vi "WheeTrometerChrom_2.vi"() -> ()   [LabVIEW 2020]
uses:
  <vilib>/Analysis/baseanly.llb/Mean (DBL).vi
  WheeChromGlobals.vi
  <vilib>/Instr/_visa.llb/VISA Configure Serial Port (Instr).vi
  <vilib>/Platform/NI_3dgraph.lvlib
  <vilib>/Analysis/NI_AALBase.lvlib
panel:
  in  "Auto Find 2":bool=TRUE
  out "Connection":bool
  in  "Tab Control":enum32{"Chrom Data", "Spectrometer Settings"}(tab)=enum."Spectrometer Settings"
  in  "3D Surface":refnum<k7>(container)
  out "Latest Spectrum":cluster{"WavelengthCal":dbl[], "Array":i32[]}(graph)
  out "Chromatogram at wavelength of interest":i32[](graph)
  in  "Start":bool
  in  "Length of Chromatogram (sec)":dbl=120.0
  in  "Wavelength of Interest (nm)":dbl=500.0
  in  "Date file path":path
  out "XY Graph":cluster{"WavelengthCal":dbl[], "Array":i32[]}(graph)
  in  "Single Spec":bool
  in  "spectra to average (per spec)":dbl=1.0
  in  "pixels to average (per spec)":dbl=2.0
  in  "Intergratin time (ms) (per spec)":dbl=2.0
  in  "Initiate":bool
  out "Connected on COM port:":refnum<visa-resource-name>="COM7"
  out "A":dbl=249.12
  out "B":dbl=0.14952
  out "C":dbl=32.477
  out "+":dbl=100.0
  out "=":dbl=125.0
  in  "Auto Find":bool=TRUE
  in  "reference":refnum<visa-resource-name>
  # "f = sin(pi*i/sizeOfdata);\n   wavelengthI(i)= A+h*B+C*f;"
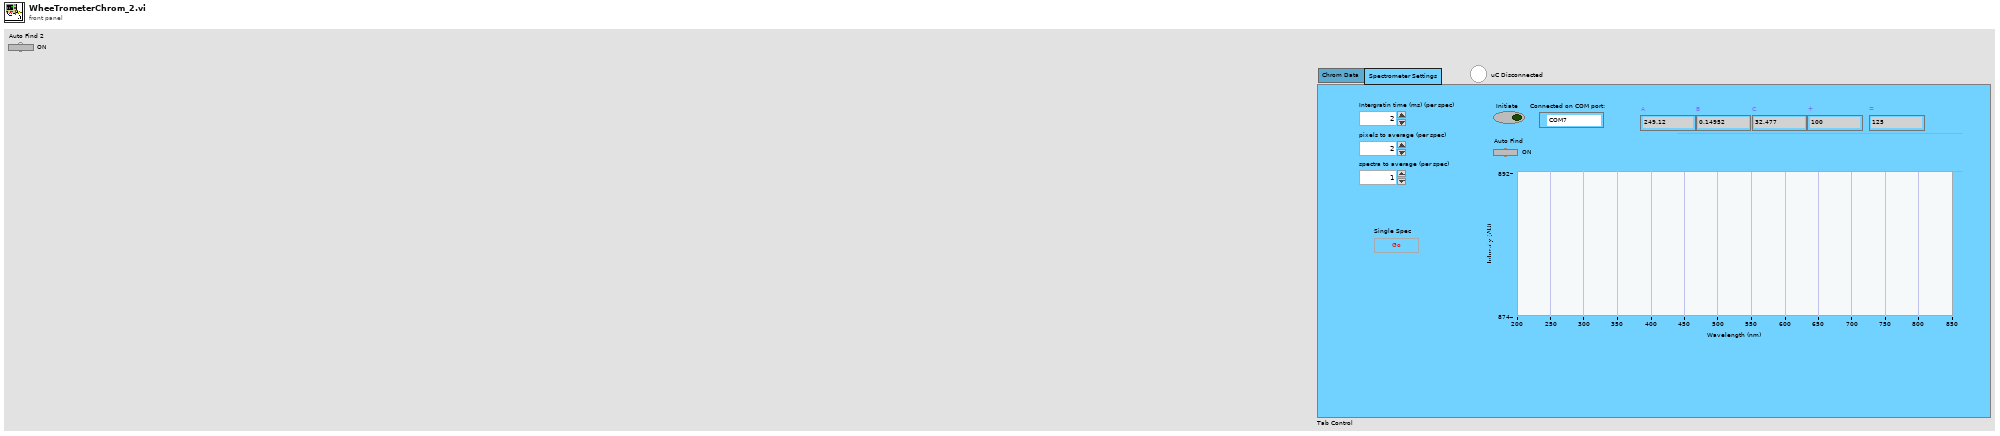
[diagram p1: front panel]
types:
  T1 = enum16{"open", "replace", "create", "open or create", "replace or create", "replace or create with confirmation"}
  T2 = enum16{"open", "open or create", "create or replace", "create", "open (read-only)"}
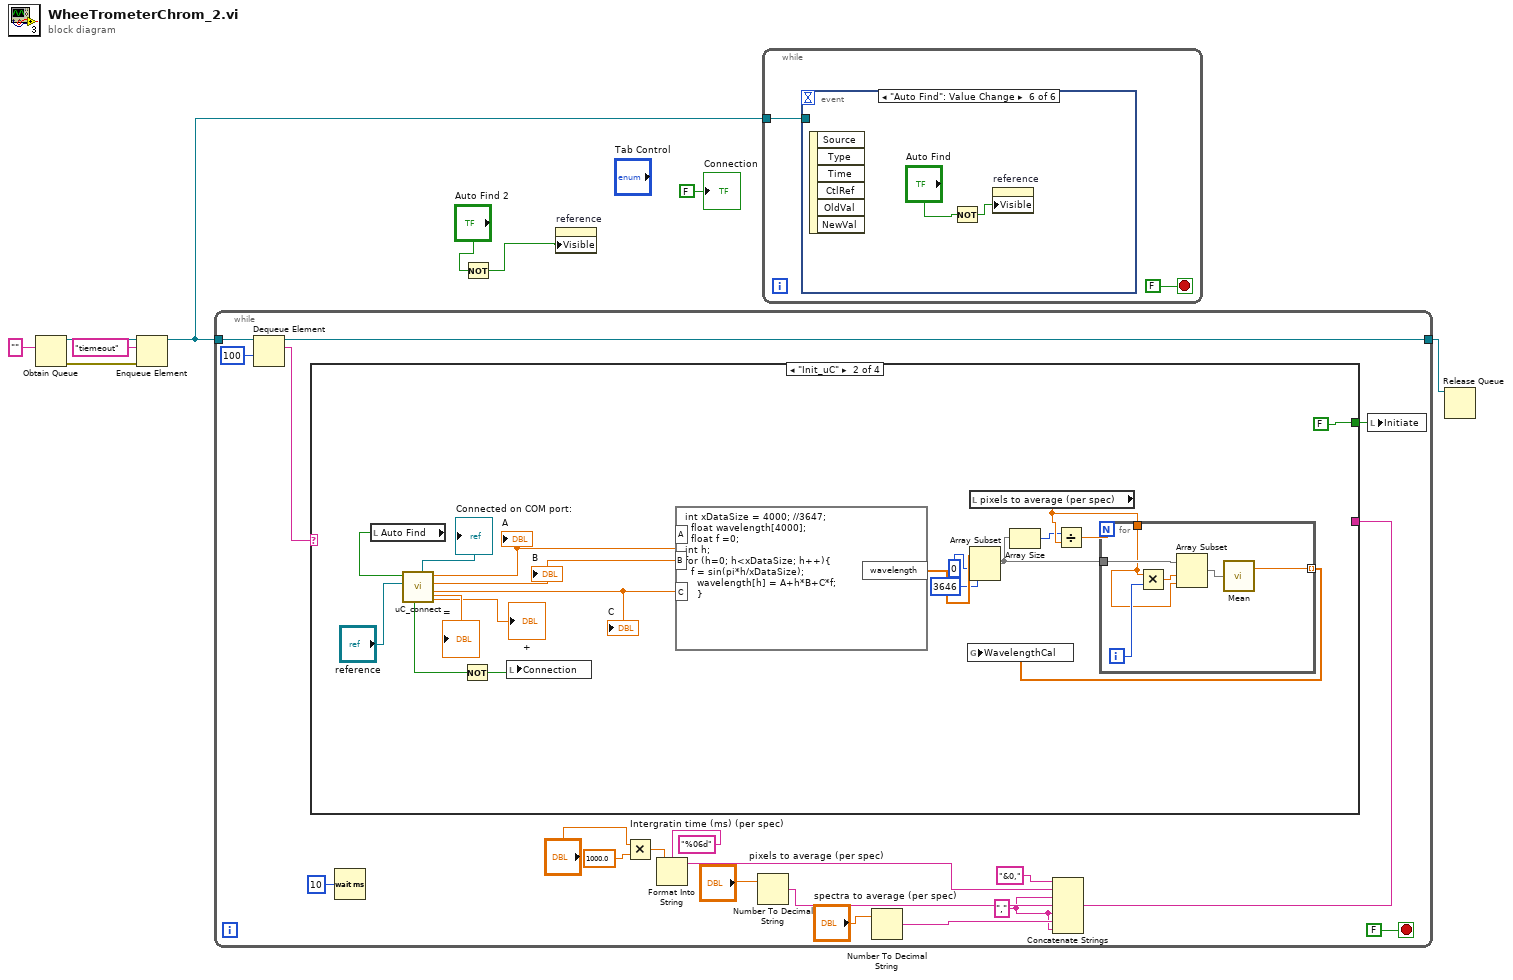
[diagram p0: block diagram]
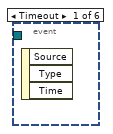
[diagram p2: hidden frame]
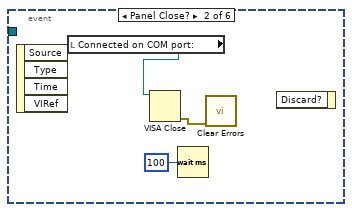
[diagram p3: hidden frame]
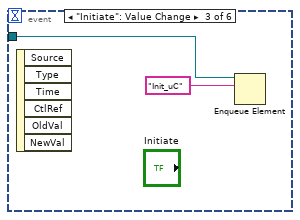
[diagram p4: hidden frame]
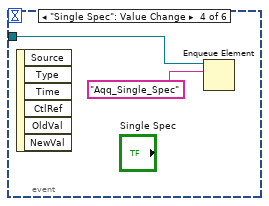
[diagram p5: hidden frame]
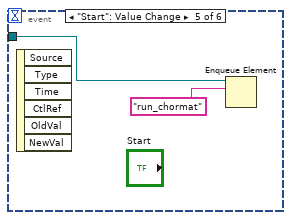
[diagram p6: hidden frame]
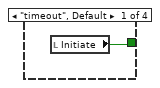
[diagram p7: hidden frame]
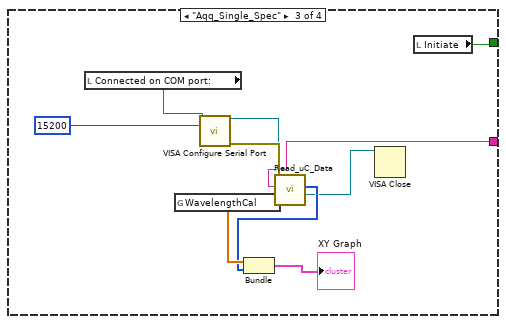
[diagram p8: hidden frame]
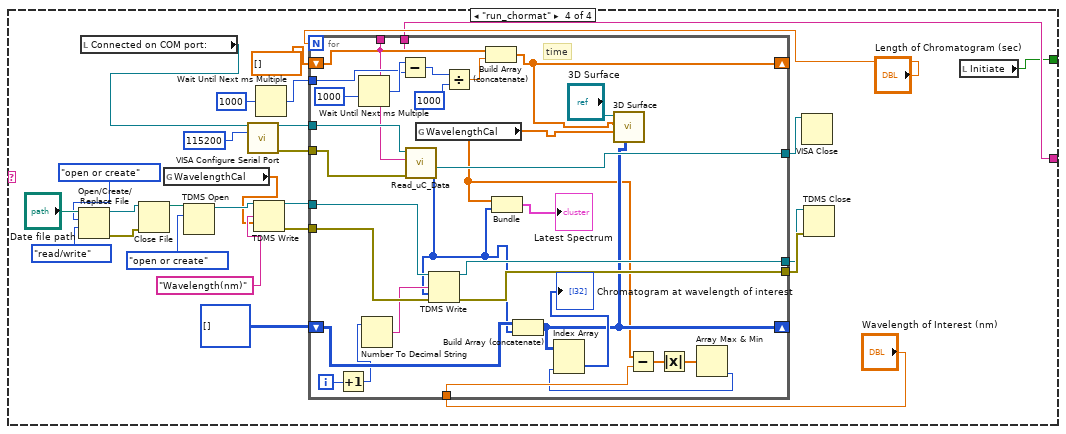
[diagram p9: hidden frame]
diagram:
  n1 = Obtain Queue(element data type="") -> (queue out=w7:refnum<queue>, error out=w5:errorcluster)  [unwired: 4 in, 1 out]
  n2 = Enqueue Element(queue=w7, element="tiemeout", error in (no error)=w5) -> (queue out=w3:refnum<queue>)  [unwired: 1 in, 2 out]
  n3 = while {
    tunnel: w3 -> [w27]
    tunnel: [w26] -> w4
    stop <- FALSE stop-if-true
    w15 = "," ("string")
    n4 = Dequeue Element(queue=w27, timeout in ms (-1)=100) -> (queue out=w26:refnum<queue>, element=w25:string)  [unwired: 1 in, 2 out]
    n5 = Wait (ms)(milliseconds to wait=u32 10) -> ()  [unwired: 1 out]
    n6 = Multiply(x="Intergratin time (ms) (per spec)", y=1000.0) -> (x*y=w17:dbl)
    n7 = Format Into String(format string="%06d", w17) -> (resulting string=w21:string)  [unwired: 2 in, 1 out]
    n8 = Number To Decimal String(number="pixels to average (per spec)") -> (decimal integer string=w22:string)  [unwired: 1 in]
    n9 = Number To Decimal String(number="spectra to average (per spec)") -> (decimal integer string=w23:string)  [unwired: 1 in]
    n10 = Concatenate Strings("&0," ("string"), w21, w15, w22, w15, w23, w15) -> (w12:string)
    n11 = case shown="\"Init_uC\"" w25 {
      tunnel: w12 -> [_ _ w57 w71]
      tunnel: [w29 FALSE ("Initiate") w55 w70] -> w10
      frame "timeout", Default {
        n12 = local read "Initiate"() -> (w29:bool)
      }
      frame "Init_uC" {
        n13 = local read "Auto Find"() -> (w32:bool)
        n14 = call "uC_connect.vi"("reference"="reference", "find port"=w32) -> ("+"=→"+":dbl, "C"=w39:dbl, "B"=w38:dbl, "A"=w37:dbl, "="=→"=":dbl, "VISA resource name out"=→"Connected on COM port:":refnum<visa-resource-name>, "status"=w48:bool)  [unwired: 2 in, 1 out]
        "A" <- w37
        "B" <- w38
        "C" <- w39
        n15 = Not(x=w48) -> (.not. x?=w47:bool)
        n16 = local write "Connection"(w47) -> ()
        n17 = formula code="int xDataSize = 4000; //3647;                \n  float wavelength[4000];\n  float f =0;\nint h;\nfor (h=0; h<xDataSize; h++){\n  f = sin(pi*h/xDataSize);\n    wavelength[h] = A+h*B+C*f;\n    }"("A"=w37, "B"=w38, "C"=w39) -> ("wavelength"=w40:dbl[])
        n18 = local read "pixels to average (per spec)"() -> (w44:dbl)
        n19 = Array Subset(array=w40, index=0, length=3646) -> (w43:dbl[])
        n20 = Array Size(array=w43) -> (size(s)=w41:i32)
        n21 = Divide(x=w41, y=w44) -> (x/y=w42:dbl)
        n22 = for {
          N: w42 -> [_]
          tunnel: w43 -> [w54]
          tunnel: w44 -> [w51]
          tunnel: [w49] -> w45 mode=indexing
          i -> [w52]
          n23 = Multiply(x=w51, y=w52) -> (x*y=w53:dbl)
          n24 = Array Subset(array=w54, index=w53, length=w51) -> (w50:dbl[])
          n25 = call-poly <vilib>:"Mean.vi"("X"=w50) -> ("mean"=w49:dbl)  [unwired: 1 out]
        }
        n26 = global write "WheeChromGlobals.vi" "WavelengthCal"(w45) -> ()
      }
      frame "Aqq_Single_Spec" {
        n27 = local read "Connected on COM port:"() -> (w58:refnum<visa-resource-name>)
        n28 = global read "WheeChromGlobals.vi" "WavelengthCal"() -> (w64:dbl[])
        n29 = call-poly "VISA Configure Serial Port"("VISA resource name"=w58, "baud rate (9600)"=u32 15200) -> ("VISA resource name out"=w59:refnum<visa-resource-name>, "error out"=w60:errorcluster)  [unwired: 12 in]
        n30 = call "Read_uC_Data.vi"("error in (no error)"=w60, "String"=w57, "VISA Refnum in"=w59) -> ("VISA Refnum in 2"=w61:refnum<visa-resource-name>, "Array"=w62:i32[])  [unwired: 6 in, 1 out]
        n31 = Bundle("WavelengthCal"=w64, "Array"=w62) -> (→"XY Graph":cluster{"WavelengthCal":dbl[], "Array":i32[]})  [unwired: 1 in]
        n32 = VISA Close(VISA resource name=w61) -> ()  [unwired: 1 in, 1 out]
        n33 = local read "Initiate"() -> (w55:bool)
      }
      frame "run_chormat" {
        n34 = Open/Create/Replace File(file path (use dialog)="Date file path", operation (0:open)=T1."open or create", access (0:read/write)=enum16{"read/write", "read-only", "write-only"}."read/write") -> (refnum out=w87:refnum<file>, error out=w86:errorcluster)  [unwired: 3 in, 1 out]
        n35 = local read "Connected on COM port:"() -> (w90:refnum<visa-resource-name>)
        n36 = Close File(refnum=w87, error in=w86) -> (path=w88:path)  [unwired: 1 out]
        n37 = global read "WheeChromGlobals.vi" "WavelengthCal"() -> (w65:dbl[])
        n38 = TDMS Open(10:T2."open or create" ("operation (0:open)"), 11:w88) -> (3:w67:refnum<k34>)  [unwired: 5 in, 1 out]
        n39 = call-poly "VISA Configure Serial Port"("VISA resource name"=w90, "baud rate (9600)"=u32 115200) -> ("VISA resource name out"=w81:refnum<visa-resource-name>, "error out"=w82:errorcluster)  [unwired: 12 in]
        n40 = TDMS Write(0:w67, 7:"Wavelength(nm)", 9:w65) -> (4:w68:refnum<k34>, 15:w69:errorcluster)  [unwired: 3 in, 2 out]
        n41 = Wait Until Next ms Multiple(millisecond multiple=u32 1000) -> (millisecond timer value=w91:u32)
        n42 = for {
          N: "Length of Chromatogram (sec)" -> [_]
          tunnel: w81 -> [w115]
          tunnel: w82 -> [w114]
          tunnel: [w94] -> _
          shift-right: [w101] -> _
          shift-left: i32[][] [] -> [w120]
          tunnel: "Wavelength of Interest (nm)" -> [w97]
          shift-right: [w100] -> _
          shift-left: dbl[] [] -> [w116]
          tunnel: [w113] -> w83
          tunnel: [w112] -> w84
          tunnel: [w111] -> w85
          tunnel: w69 -> [w110]
          tunnel: w68 -> [w109]
          tunnel: w91 -> [w103]
          tunnel: w71 -> [w94]
          i -> [w93]
          # "time"
          n43 = Increment(x=w93) -> (x+1=w92:i32)
          n44 = Wait Until Next ms Multiple(millisecond multiple=u32 1000) -> (millisecond timer value=w104:u32)
          n45 = Number To Decimal String(number=w92) -> (decimal integer string=w108:string)  [unwired: 1 in]
          n46 = Subtract(x=w104, y=w103) -> (x-y=w105:u32)
          n47 = call "Read_uC_Data.vi"("error in (no error)"=w114, "String"=w94, "VISA Refnum in"=w115) -> ("VISA Refnum in 2"=w113:refnum<visa-resource-name>, "Array"=w106:i32[])  [unwired: 6 in, 1 out]
          n48 = global read "WheeChromGlobals.vi" "WavelengthCal"() -> (w96:dbl[])
          n49 = TDMS Write(0:w109, 7:w108, 9:w106, 11:w110) -> (4:w112:refnum<k34>, 15:w111:errorcluster)  [unwired: 2 in, 2 out]
          n50 = Divide(x=w105, y=u32 1000) -> (x/y=w117:dbl)
          n51 = Build Array (concatenate)(w116, w117) -> (w100:dbl[])
          n52 = Bundle("WavelengthCal"=w96, "Array"=w106) -> (→"Latest Spectrum":cluster{"WavelengthCal":dbl[], "Array":i32[]})  [unwired: 1 in]
          n53 = Build Array (concatenate)(w120, w106) -> (w101:i32[][])
          n54 = call <vilib>:"3D Surface.vi"("z matrix"=w101, "y vector"=w96, "x vector"=w100, "3D graph"="3D Surface") -> ()  [unwired: 6 in, 2 out]
          n55 = Subtract(x=w96, y=w97) -> (x-y=w99:dbl[])
          n56 = Absolute Value(x=w99) -> (abs(x)=w98:dbl[])
          n57 = Array Max & Min(array=w98) -> (min index (indices)=w95:i32)  [unwired: 3 out]
          n58 = Index Array(array=w101, index (col)=w95) -> (element=→"Chromatogram at wavelength of interest":i32[])  [unwired: 1 in]
        }
        n59 = VISA Close(VISA resource name=w83) -> ()  [unwired: 1 in, 1 out]
        n60 = TDMS Close(8:w85, 11:w84) -> ()  [unwired: 2 out]
        n61 = local read "Initiate"() -> (w70:bool)
      }
    }
    n62 = local write "Initiate"(w10) -> ()
  }
  n63 = Not(x="Auto Find 2") -> (.not. x?=w1:bool)
  n64 = property on="reference" class="VISAName"("Visible"=w1) -> ()  [unwired: 2 in, 2 out]
  n65 = while {
    tunnel: w3 -> [w123]
    stop <- FALSE stop-if-true
    n66 = event shown="[5] \"Auto Find\": Value Change" {
      selector: _ -> [_ _ _ _ _ _]
      dyn-events: _ -> [_ _ _ _ _ _]
      timeout: _ -> [_ _ _ _ _ _]
      tunnel: w123 -> [_ _ w127 w129 w131 _]
      event Timeout {
        n67 = event-data() -> ()  [unwired: 1 in, 3 out]
      }
      event Panel Close? {
        n68 = event-data() -> ()  [unwired: 1 in, 4 out]
        n69 = local read "Connected on COM port:"() -> (w126:refnum<visa-resource-name>)
        n70 = VISA Close(VISA resource name=w126) -> (error out=w125:errorcluster)  [unwired: 1 in]
        n71 = Wait (ms)(milliseconds to wait=u32 100) -> ()  [unwired: 1 out]
        n72 = call <vilib>:"Clear Errors.vi"("error in (no error)"=w125) -> ()  [unwired: 5 in, 2 out]
        n73 = event-data() -> ()  [unwired: 2 in, 1 out]
      }
      event "Initiate": Value Change {
        n74 = event-data() -> ()  [unwired: 1 in, 6 out]
        n75 = Enqueue Element(queue=w127, element="Init_uC") -> ()  [unwired: 2 in, 3 out]
      }
      event "Single Spec": Value Change {
        n76 = event-data() -> ()  [unwired: 1 in, 6 out]
        n77 = Enqueue Element(queue=w129, element="Aqq_Single_Spec") -> ()  [unwired: 2 in, 3 out]
      }
      event "Start": Value Change {
        n78 = event-data() -> ()  [unwired: 1 in, 6 out]
        n79 = Enqueue Element(queue=w131, element="run_chormat") -> ()  [unwired: 2 in, 3 out]
      }
      event "Auto Find": Value Change {
        n80 = event-data() -> ()  [unwired: 1 in, 6 out]
        n81 = Not(x="Auto Find") -> (.not. x?=w133:bool)
        n82 = property on="reference" class="VISAName"("Visible"=w133) -> ()  [unwired: 2 in, 2 out]
      }
    }
  }
  n83 = Release Queue(queue=w4) -> ()  [unwired: 2 in, 3 out]
  "Connection" <- FALSE ("Connection")
